vi "Main.vi"(11 "Module Admin":refnum<class "Delacor_lib_QMH_Module Admin.lvclass">) -> ()   [LabVIEW 2021, in "Database.lvlib"]
doc: "This template is based off of the Queued Message Handler design pattern and the Queued Message Handler project template that ships with LabVIEW.\n\nThe main difference is that the queue is private to this module and communication between modules is performed via Broadcast and Request events.\n\nRequest events are wrapped in public API methods and are handled in the Event Handling Loop (EHL) of this VI. Any module can register for Broadcast events sent by this module. The EHL generates messages based on user interface actions.\n\nThe Message Handling Loop (MHL) processes messages generated by the EHL, or by other messages. The messages are string values, so new messages can be added easily to the Message Cases case structure in the MHL. Each message cluster can also provide an optional value for Message Data, which is a variant that can be converted to whatever message-specific data is required.\n_____\nBased on DQMH Project Template 6.1.0.94."
uses:
  Database.lvlib
  <vilib>/Delacor/Delacor QMH/Libraries/Module Admin_class/Delacor_lib_QMH_Module Admin.lvclass
  Class/Access/Access.lvclass
  C:/repository/common_ATE/Libraries/Database/Class/DB/DB.lvclass
  Class/DB/DB.lvclass
  Module Data--cluster.ctl
  <vilib>/Delacor/Delacor QMH/Libraries/Message Queue_class/Delacor_lib_QMH_Message Queue.lvclass/Delacor_lib_QMH_Message Queue.ctl
  Stop Argument--cluster.ctl
  <vilib>/Delacor/Delacor QMH/Libraries/Module Admin_class/Delacor_lib_QMH_Module Admin.lvclass/Delacor_lib_QMH_Module Admin.ctl
  REQ Add User Argument--cluster.ctl
  Class/DB/Credential.ctl
  REQ Check Credential Argument--cluster.ctl
  REQ Check Credential (Reply Payload)--cluster.ctl
  REQ Delete User Argument--cluster.ctl
  REQ Update User Details Argument--cluster.ctl
  Class/DB/Update Credential.ctl
  REQ List Table Argument--cluster.ctl
  REQ List Table (Reply Payload)--cluster.ctl
  REQ Delete Table Data Argument--cluster.ctl
  REQ Save DB Record Data Argument--cluster.ctl
  REQ Save Test Data Argument--cluster.ctl
  REQ Load Test Data Argument--cluster.ctl
  REQ Load Test Data (Reply Payload)--cluster.ctl
  REQ Get Username Argument--cluster.ctl
  REQ Get Username (Reply Payload)--cluster.ctl
  REQ Close DB Ref Argument--cluster.ctl
  <vilib>/Utility/miscctls.llb/LVPointTypeDef.ctl
  <vilib>/Delacor/Delacor QMH/Libraries/Message Queue_class/Delacor_lib_QMH_Enqueue Message (Single).vi
  <vilib>/Delacor/Delacor QMH/Libraries/Module Admin_class/Delacor_lib_QMH_Get External Launch.vi
  <vilib>/Utility/error.llb/Error Cluster From Error Code.vi
  <vilib>/ErrorRing/Error Ring.xnode
  <vilib>/Delacor/Delacor QMH/Libraries/Message Queue_class/Delacor_lib_QMH_Message Queue.lvclass
panel:
  out "error out":errorcluster
  out "Status":string
  in  "Simulate MHL Error":bool
  in  "Simulate EHL Error":bool
  # "Other QMH Modules communicate with this Module via its Public API (wrappers for its Request Events).\n\nThis Module communicates with other Modules via its Broadcast Events.\nAny module that wants to get these messages, just registers for this module's Broadcast events."
  # "This template is for the Delacor Modified Queued Message Handler design pattern.\n\nSee the block diagram for more information on how to use this template."
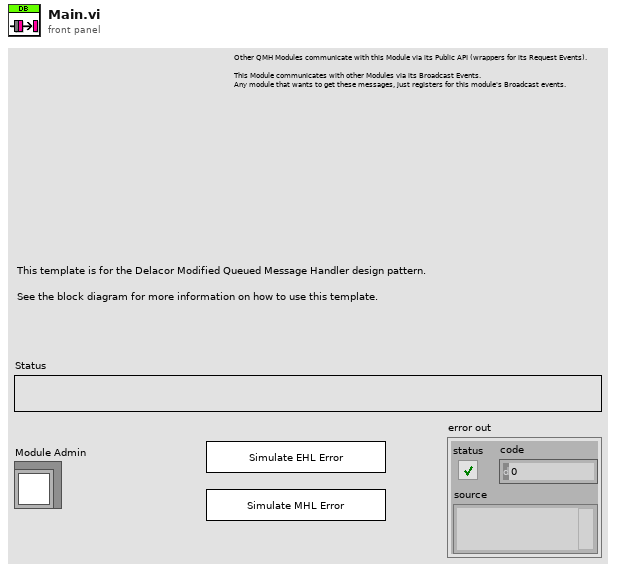
[diagram p1: front panel]
types:
  T1 = typedef "Database.lvlib/Request Events--cluster.ctl" = cluster{"Stop Module":refnum<user-event>, "Show Panel":refnum<user-event>, "Hide Panel":refnum<user-event>, "Get Module Execution Status":refnum<user-event>, "Show Diagram":refnum<user-event>, "REQ Add User":refnum<user-event>, "REQ Check Credential":refnum<user-event>, "REQ Delete User":refnum<user-event>, "REQ Update User Details":refnum<user-event>, "REQ List Table":refnum<user-event>, "REQ Delete Table Data":refnum<user-event>, "REQ Save DB Record Data":refnum<user-event>, "REQ Save Test Data":refnum<user-event>, "REQ Load Test Data":refnum<user-event>, "REQ Get Username":refnum<user-event>, "REQ Close DB Ref":refnum<user-event>}
  T2 = typedef "Database.lvlib/Module Data--cluster.ctl" = cluster{"Status":string, "DB.lvclass":refnum<class "DB.lvclass">}
  T3 = enum32{"invalid lock state", "Not Locked", "Locked (No Password)", "Password-protected"}
  T4 = typedef "Database.lvlib/Stop Argument--cluster.ctl" = cluster{"Origin":string, "Exit via Stop Module Req?":bool, "Wait for Module to stop?":bool}
  T5 = typedef "Database.lvlib/REQ Add User Argument--cluster.ctl" = cluster{"Credential":T6}
  T6 = typedef "Database.lvlib/Credential.ctl" = cluster{"User Level":enum16{"Administrator", "Engineer", "Operator"}, "User Name":string, "Password":string}
  T7 = typedef "Database.lvlib/REQ Check Credential Argument--cluster.ctl" = cluster{"Credential":T6, "Wait Notifier":refnum<notifier>, "wait for reply":bool}
  T8 = typedef "Database.lvlib/REQ Delete User Argument--cluster.ctl" = cluster{"Credential":T6}
  T9 = typedef "Database.lvlib/REQ Update User Details Argument--cluster.ctl" = cluster{"Update Credential":T10}
  T10 = typedef "Database.lvlib/Update Credential.ctl" = cluster{"User Level":enum16{"Administrator", "Engineer", "Operator"}, "User Name":string, "Old Password":string, "New Password":string}
  T11 = typedef "Database.lvlib/REQ List Table Argument--cluster.ctl" = cluster{"Table?":bool, "Wait Notifier":refnum<notifier>, "wait for reply":bool}
  T12 = typedef "Database.lvlib/REQ Delete Table Data Argument--cluster.ctl" = cluster{"Table name":string}
  T13 = typedef "Database.lvlib/REQ Save DB Record Data Argument--cluster.ctl" = cluster{"Boolean":bool}
  T14 = typedef "Database.lvlib/REQ Save Test Data Argument--cluster.ctl" = cluster{"Test Data":string[]}
  T15 = typedef "Database.lvlib/REQ Load Test Data Argument--cluster.ctl" = cluster{"From":timestamp, "To":timestamp, "Wait Notifier":refnum<notifier>, "wait for reply":bool}
  T16 = typedef "Database.lvlib/REQ Get Username Argument--cluster.ctl" = cluster{"User Level":enum16{"Administrator", "Engineer", "Operator"}, "Wait Notifier":refnum<notifier>, "wait for reply":bool}
  T17 = typedef "Database.lvlib/REQ Close DB Ref Argument--cluster.ctl" = cluster{"Boolean":bool}
  T18 = typedef "LVPointTypeDef.ctl" = cluster{"Horizontal":i16, "Vertical":i16}
  T19 = enum32{"Invalid", "Standard", "Closed", "Hidden", "Minimized", "Maximized"}
  T20 = typedef "Database.lvlib/REQ Check Credential (Reply Payload)--cluster.ctl" = cluster{"Match?":bool, "error":errorcluster}
  T21 = typedef "Database.lvlib/REQ List Table (Reply Payload)--cluster.ctl" = cluster{"List Table":string[], "error":errorcluster}
  T22 = typedef "Database.lvlib/REQ Load Test Data (Reply Payload)--cluster.ctl" = cluster{"Test Data":string[][], "error":errorcluster}
  T23 = typedef "Database.lvlib/REQ Get Username (Reply Payload)--cluster.ctl" = cluster{"Username":string[], "error":errorcluster}
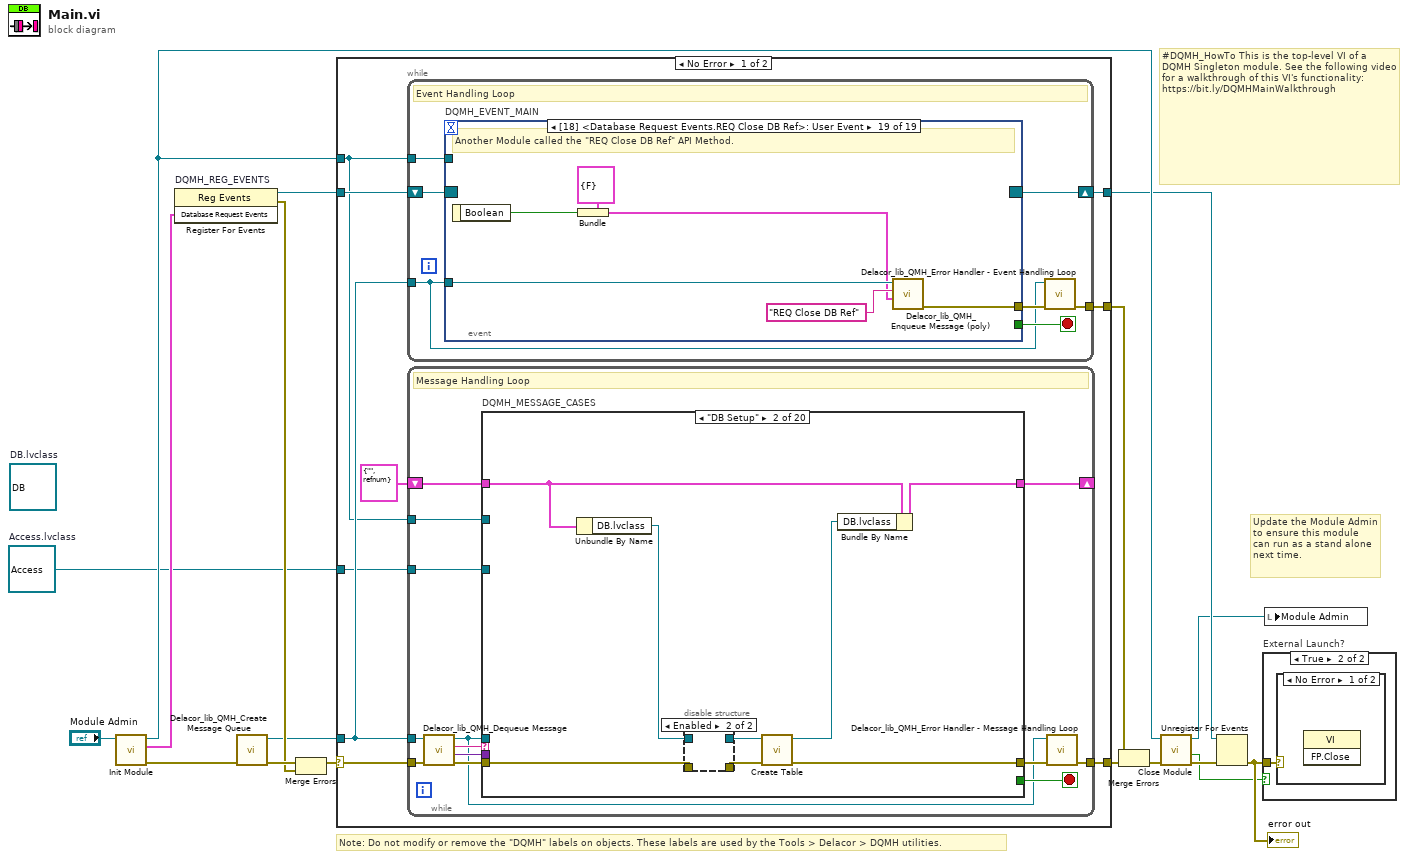
[diagram p0: block diagram]
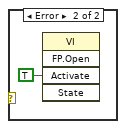
[diagram p3: hidden frame]
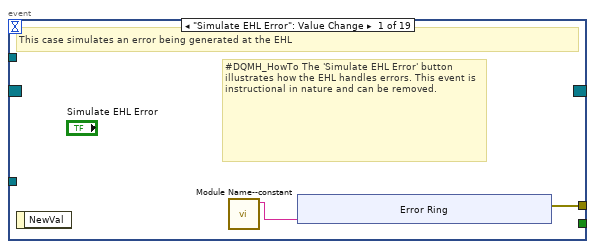
[diagram p4: hidden frame]
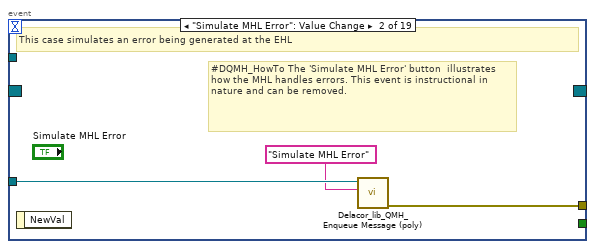
[diagram p5: hidden frame]
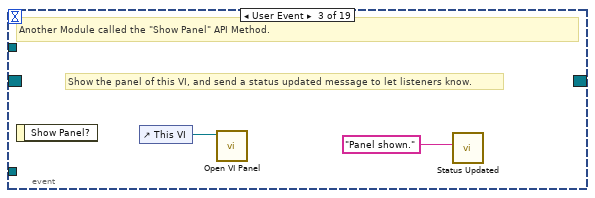
[diagram p6: hidden frame]
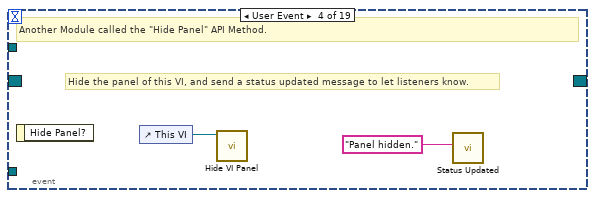
[diagram p7: hidden frame]
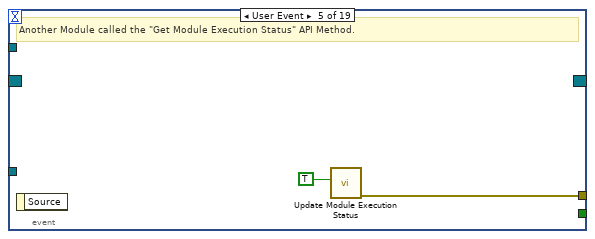
[diagram p8: hidden frame]
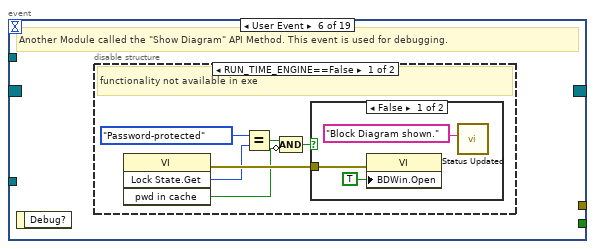
[diagram p9: hidden frame]
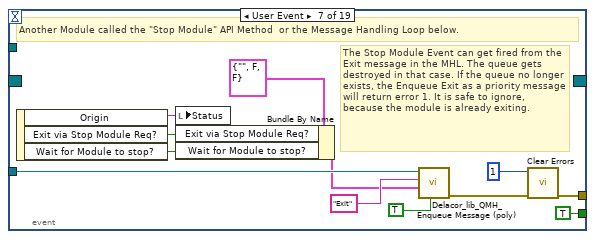
[diagram p12: hidden frame]
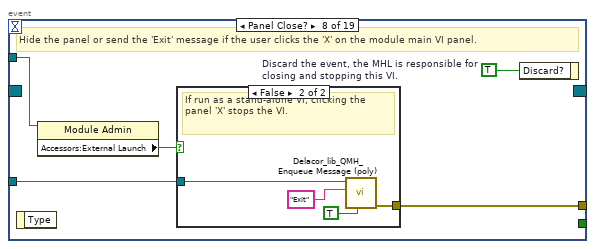
[diagram p13: hidden frame]
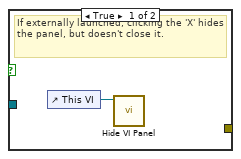
[diagram p14: hidden frame]
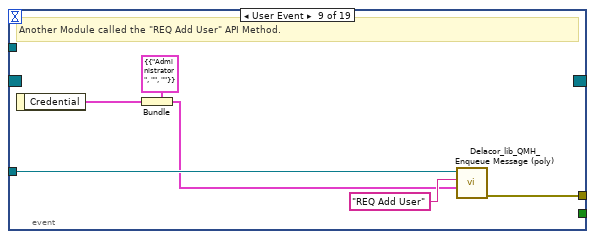
[diagram p15: hidden frame]
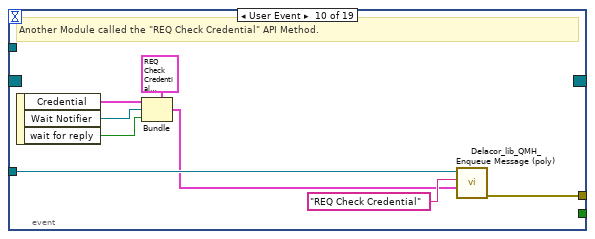
[diagram p16: hidden frame]
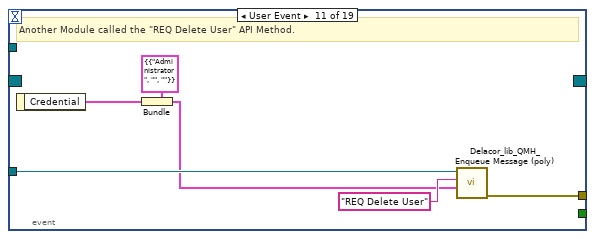
[diagram p17: hidden frame]
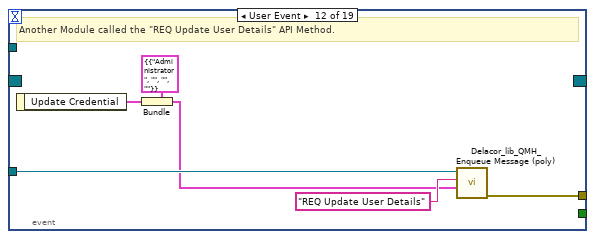
[diagram p18: hidden frame]
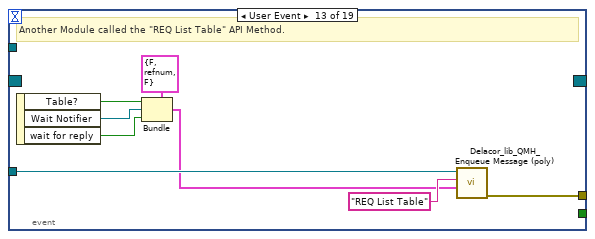
[diagram p19: hidden frame]
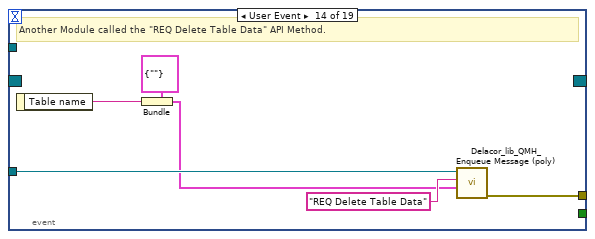
[diagram p20: hidden frame]
diagram:
  w1 = refnum<class "Access.lvclass"> refnum  # Access.lvclass
  (unwired) refnum<class "DB.lvclass"> refnum  # DB.lvclass
  # "#DQMH_HowTo This is the top-level VI of a DQMH Singleton module. See the following video for a walkthrough of this VI's functionality: https://bit.ly/DQMHMainWalkthrough"
  # "Note: Do not modify or remove the \"DQMH\" labels on objects. These labels are used by the Tools > Delacor > DQMH utilities."
  # "Update the Module Admin to ensure this module can run as a stand alone next time."
  n1 = call "Init Module.vi"("Singleton Module Admin in"="Module Admin") -> ("error out"=w17:errorcluster, "Database Request Events"=w6:T1, "Singleton Module Admin out"=w9:refnum<class "Delacor_lib_QMH_Module Admin.lvclass">)  [unwired: 8 in]
  n2 = register-events "DQMH_REG_EVENTS"(w6) -> (reference out=w7:refnum<event-registration>, error out=w10:errorcluster)  [unwired: 2 in]
  n3 = call <vilib>:"Delacor_lib_QMH_Create Message Queue.vi"("error in"=w17) -> ("error out"=w12:errorcluster, "Message Queue"=w5:refnum<class "Delacor_lib_QMH_Message Queue.lvclass">)  [unwired: 9 in]
  n4 = Merge Errors(w12, w10) -> (w11:errorcluster)
  n5 = case shown="No Error" w11 {
    selector: w11 -> [w25 w426]
    tunnel: [w27 w425] -> w18
    tunnel: [w24 w431] -> w8
    tunnel: w7 -> [w22 w431]
    tunnel: w5 -> [w21 w424]
    tunnel: [w26 _] -> w15
    tunnel: w9 -> [w20 w427]
    tunnel: w1 -> [w19 _]
    frame No Error {
      n6 = while {
        tunnel: w21 -> [w28]
        shift-right: [w31] -> w24
        shift-left: w22 -> [w32]
        tunnel: [w33] -> w26
        tunnel: w20 -> [w29]
        stop <- w30 stop-if-true
        # "Event Handling Loop"
        n7 = event "DQMH_EVENT_MAIN" shown="[18] <Database Request Events.REQ Close DB Ref>: User Event" {
          selector: w32 -> [_ _ _ _ _ _ _ _ _ _ _ _ _ _ _ _ _ _ _]
          dyn-events: [_ _ _ _ _ _ _ _ _ _ _ _ _ _ _ _ _ _ _] -> w31
          timeout: _ -> [_ _ _ _ _ _ _ _ _ _ _ _ _ _ _ _ _ _ _]
          tunnel: [_ _ _ _ _ _ TRUE ("Discard?") _ _ _ _ _ _ _ _ _ _ _ _] -> w30
          tunnel: w28 -> [_ w45 _ _ _ _ w69 w76 w89 w97 w103 w109 w117 w123 w129 w135 w144 w152 w158]
          tunnel: [w36 w46 _ _ w52 _ w72 w78 w85 w90 w98 w104 w110 w118 w124 w130 w136 w145 w153] -> w34
          tunnel: w29 -> [_ _ _ _ _ _ _ w75 _ _ _ _ _ _ _ _ _ _ _]
          event "Simulate EHL Error": Value Change {
            # "#DQMH_HowTo The 'Simulate EHL Error' button  illustrates how the EHL handles errors. This event is instructional in nature and can be removed."
            # "This case simulates an error being generated at the EHL"
            n8 = event-data() -> ()  [unwired: 1 in, 1 out]
            n9 = call "Module Name--constant.vi"() -> ("Module Name"=w35:string)  [unwired: 11 in]
            n10 = xnode "Error Ring"("parameter 0"=w35) -> ("error out"=w36:errorcluster)
          }
          event "Simulate MHL Error": Value Change {
            # "#DQMH_HowTo The 'Simulate MHL Error' button  illustrates how the MHL handles errors. This event is instructional in nature and can be removed."
            # "This case simulates an error being generated at the EHL"
            n11 = event-data() -> ()  [unwired: 1 in, 1 out]
            n12 = call-poly <vilib>:"Delacor_lib_QMH_Enqueue Message (poly).vi"("Message"="Simulate MHL Error", "Message Queue in"=w45) -> ("error out"=w46:errorcluster)  [unwired: 8 in, 1 out]
          }
          event User Event {
            # "Show the panel of this VI, and send a status updated message to let listeners know."
            # "Another Module called the \"Show Panel\" API Method."
            n13 = event-data() -> ()  [unwired: 1 in, 1 out]
            n14 = control-ref of="This VI"() -> (w48:refnum<vi>)
            n15 = call "Open VI Panel.vi"("VI"=w48) -> ()  [unwired: 10 in, 1 out]
            n16 = call "Status Updated.vi"("Status"="Panel shown." ("format string")) -> ()  [unwired: 10 in, 1 out]
          }
          event User Event {
            # "Hide the panel of this VI, and send a status updated message to let listeners know."
            # "Another Module called the \"Hide Panel\" API Method."
            n17 = event-data() -> ()  [unwired: 1 in, 1 out]
            n18 = control-ref of="This VI"() -> (w50:refnum<vi>)
            n19 = call "Hide VI Panel.vi"("VI"=w50) -> ()  [unwired: 10 in, 1 out]
            n20 = call "Status Updated.vi"("Status"="Panel hidden." ("format string")) -> ()  [unwired: 10 in, 1 out]
          }
          event User Event {
            # "Another Module called the \"Get Module Execution Status\" API Method."
            n21 = event-data() -> ()  [unwired: 1 in, 1 out]
            n22 = call "Update Module Execution Status.vi"("Running?"=TRUE) -> ("error out"=w52:errorcluster)  [unwired: 10 in]
          }
          event User Event {
            # "Another Module called the \"Show Diagram\" API Method. This event is used for debugging."
            n23 = event-data() -> ()  [unwired: 1 in, 1 out]
            n24 = disable-structure shown="RUN_TIME_ENGINE==False" {
              frame condition #0 (active) {
                # "functionality not available in exe"
                n25 = invoke class="VI" method="Lock State.Get"() -> (error out=w58:errorcluster, "Get Lock State"=w57:T3, "pwd in cache"=w54:bool)  [unwired: 4 in, 1 out]
                n26 = Equal?(x=T3."Password-protected", y=w57) -> (x = y?=w55:bool)
                n27 = Compound Arithmetic op=AND(w55, invert w54) -> (w53:bool)
                n28 = case shown="False" w53 {
                  tunnel: w58 -> [w61 _]
                  frame False {
                    n29 = property class="VI"(error in=w61, "BDWin.Open"=TRUE ("Block Diagram Window:Open")) -> ()  [unwired: 1 in, 2 out]
                    n30 = call "Status Updated.vi"("Status"="Block Diagram shown." ("format string")) -> ()  [unwired: 10 in, 1 out]
                  }
                  frame True {
                    # "Password-protected VI, and the password is not in the cache. Do not show the diagram."
                  }
                }
              }
              frame condition #1 {
              }
            }
          }
          event User Event {
            # "The Stop Module Event can get fired from the Exit message in the MHL. The queue gets destroyed in that case. If the queue no longer exists, the Enqueue Exit as a priority message will return error 1. It is safe to ignore, because the module is already exiting."
            # "Another Module called the \"Stop Module\" API Method  or the Message Handling Loop below."
            n31 = event-data() -> ("Origin"=w68:string, "Exit via Stop Module Req?"=w64:bool, "Wait for Module to stop?"=w63:bool)  [unwired: 1 in]
            n32 = local write "Status"(w68) -> ()
            n33 = Bundle By Name(cluster=T4 {"Origin"="", "Exit via Stop Module Req?"=FALSE, "Wait for Module to stop?"=FALSE} ("Stop Argument"), "Exit via Stop Module Req?"=w64, "Wait for Module to stop?"=w63) -> (w62:T4)
            n34 = call-poly <vilib>:"Delacor_lib_QMH_Enqueue Message (poly).vi"("Priority Message? (F)"=TRUE, "Message Data"=w62, "Message"="Exit", "Message Queue in"=w69) -> ("error out"=w73:errorcluster)  [unwired: 6 in, 1 out]
            n35 = call <vilib>:"Clear Errors.vi"("error in (no error)"=w73, "specific error code to clear (0: all)"=1) -> ("error out"=w72:errorcluster)  [unwired: 4 in, 1 out]
          }
          event Panel Close? {
            w77 = TRUE  # Discard the event, the MHL is responsible for closing and stopping this VI.
            # "Hide the panel or send the 'Exit' message if the user clicks the 'X' on the module main VI panel."
            n36 = event-data() -> ()  [unwired: 1 in, 1 out]
            n37 = property class="Module Admin"(reference=w75) -> ("Accessors:External Launch"=w74:bool)  [unwired: 1 in, 2 out]
            n38 = case shown="False" w74 {
              tunnel: w76 -> [_ w82]
              tunnel: [_ w83] -> w78
              frame True {
                # "If externally launched, clicking the 'X' hides the panel, but doesn't close it."
                n39 = control-ref of="This VI"() -> (w79:refnum<vi>)
                n40 = call "Hide VI Panel.vi"("VI"=w79) -> ()  [unwired: 10 in, 1 out]
              }
              frame False {
                # "If run as a stand-alone VI, clicking the panel 'X' stops the VI."
                n41 = call-poly <vilib>:"Delacor_lib_QMH_Enqueue Message (poly).vi"("Priority Message? (F)"=TRUE, "Message"="Exit", "Message Queue in"=w82) -> ("error out"=w83:errorcluster)  [unwired: 7 in, 1 out]
              }
            }
            n42 = event-data("Discard?"=w77) -> ()  [unwired: 1 in, 1 out]
          }
          event User Event {
            # "Another Module called the \"REQ Add User\" API Method."
            n43 = event-data() -> ("Credential"=w84:T6)  [unwired: 1 in]
            n44 = Bundle(cluster=T5 {"Credential"={"User Level"=enum."Administrator", "User Name"="", "Password"=""}} ("REQ Add User Argument"), "Credential"=w84) -> (w86:T5)
            n45 = call-poly <vilib>:"Delacor_lib_QMH_Enqueue Message (poly).vi"("Message Data"=w86, "Message"="REQ Add User", "Message Queue in"=w89) -> ("error out"=w85:errorcluster)  [unwired: 7 in, 1 out]
          }
          event User Event {
            # "Another Module called the \"REQ Check Credential\" API Method."
            n46 = event-data() -> ("Credential"=w93:T6, "Wait Notifier"=w92:refnum<notifier>, "wait for reply"=w91:bool)  [unwired: 1 in]
            n47 = Bundle(cluster=T7 {"Credential"={"User Level"=enum."Administrator", "User Name"="", "Password"=""}, "Wait Notifier"=refnum, "wait for reply"=FALSE} ("REQ Check Credential Argument"), "Credential"=w93, "Wait Notifier"=w92, "wait for reply"=w91) -> (w94:T7)
            n48 = call-poly <vilib>:"Delacor_lib_QMH_Enqueue Message (poly).vi"("Message Data"=w94, "Message"="REQ Check Credential", "Message Queue in"=w97) -> ("error out"=w90:errorcluster)  [unwired: 7 in, 1 out]
          }
          event User Event {
            # "Another Module called the \"REQ Delete User\" API Method."
            n49 = event-data() -> ("Credential"=w99:T6)  [unwired: 1 in]
            n50 = Bundle(cluster=T8 {"Credential"={"User Level"=enum."Administrator", "User Name"="", "Password"=""}} ("REQ Delete User Argument"), "Credential"=w99) -> (w100:T8)
            n51 = call-poly <vilib>:"Delacor_lib_QMH_Enqueue Message (poly).vi"("Message Data"=w100, "Message"="REQ Delete User", "Message Queue in"=w103) -> ("error out"=w98:errorcluster)  [unwired: 7 in, 1 out]
          }
          event User Event {
            # "Another Module called the \"REQ Update User Details\" API Method."
            n52 = event-data() -> ("Update Credential"=w105:T10)  [unwired: 1 in]
            n53 = Bundle(cluster=T9 {"Update Credential"={"User Level"=enum."Administrator", "User Name"="", "Old Password"="", "New Password"=""}} ("REQ Update User Details Argument"), "Update Credential"=w105) -> (w106:T9)
            n54 = call-poly <vilib>:"Delacor_lib_QMH_Enqueue Message (poly).vi"("Message Data"=w106, "Message"="REQ Update User Details", "Message Queue in"=w109) -> ("error out"=w104:errorcluster)  [unwired: 7 in, 1 out]
          }
          event User Event {
            # "Another Module called the \"REQ List Table\" API Method."
            n55 = event-data() -> ("Table?"=w113:bool, "Wait Notifier"=w112:refnum<notifier>, "wait for reply"=w111:bool)  [unwired: 1 in]
            n56 = Bundle(cluster=T11 {"Table?"=FALSE, "Wait Notifier"=refnum, "wait for reply"=FALSE} ("REQ List Table Argument"), "Table?"=w113, "Wait Notifier"=w112, "wait for reply"=w111) -> (w114:T11)
            n57 = call-poly <vilib>:"Delacor_lib_QMH_Enqueue Message (poly).vi"("Message Data"=w114, "Message"="REQ List Table", "Message Queue in"=w117) -> ("error out"=w110:errorcluster)  [unwired: 7 in, 1 out]
          }
          event User Event {
            # "Another Module called the \"REQ Delete Table Data\" API Method."
            n58 = event-data() -> ("Table name"=w119:string)  [unwired: 1 in]
            n59 = Bundle(cluster=T12 {"Table name"=""} ("REQ Delete Table Data Argument"), "Table name"=w119) -> (w120:T12)
            n60 = call-poly <vilib>:"Delacor_lib_QMH_Enqueue Message (poly).vi"("Message Data"=w120, "Message"="REQ Delete Table Data", "Message Queue in"=w123) -> ("error out"=w118:errorcluster)  [unwired: 7 in, 1 out]
          }
          event User Event {
            # "Another Module called the \"REQ Save DB Record Data\" API Method."
            n61 = event-data() -> ("Boolean"=w125:bool)  [unwired: 1 in]
            n62 = Bundle(cluster=T13 {"Boolean"=FALSE} ("REQ Save DB Record Data Argument"), "Boolean"=w125) -> (w126:T13)
            n63 = call-poly <vilib>:"Delacor_lib_QMH_Enqueue Message (poly).vi"("Message Data"=w126, "Message"="REQ Save DB Record Data", "Message Queue in"=w129) -> ("error out"=w124:errorcluster)  [unwired: 7 in, 1 out]
          }
          event User Event {
            # "Another Module called the \"REQ Save Test Data\" API Method."
            n64 = event-data() -> ("Test Data"=w131:string[])  [unwired: 1 in]
            n65 = Bundle(cluster=T14 {"Test Data"=[]} ("REQ Save Test Data Argument"), "Test Data"=w131) -> (w132:T14)
            n66 = call-poly <vilib>:"Delacor_lib_QMH_Enqueue Message (poly).vi"("Message Data"=w132, "Message"="REQ Save Test Data", "Message Queue in"=w135) -> ("error out"=w130:errorcluster)  [unwired: 7 in, 1 out]
          }
          event User Event {
            # "Another Module called the \"REQ Load Test Data\" API Method."
            n67 = event-data() -> ("From"=w140:timestamp, "To"=w139:timestamp, "Wait Notifier"=w138:refnum<notifier>, "wait for reply"=w137:bool)  [unwired: 1 in]
            n68 = Bundle(cluster=T15 {"From"=timestamp(0 s since 1904-01-01), "To"=timestamp(0 s since 1904-01-01), "Wait Notifier"=refnum, "wait for reply"=FALSE} ("REQ Load Test Data Argument"), "From"=w140, "To"=w139, "Wait Notifier"=w138, "wait for reply"=w137) -> (w141:T15)
            n69 = call-poly <vilib>:"Delacor_lib_QMH_Enqueue Message (poly).vi"("Message Data"=w141, "Message"="REQ Load Test Data", "Message Queue in"=w144) -> ("error out"=w136:errorcluster)  [unwired: 7 in, 1 out]
          }
          event User Event {
            # "Another Module called the \"REQ Get Username\" API Method."
            n70 = event-data() -> ("User Level"=w148:enum16{"Administrator", "Engineer", "Operator"}, "Wait Notifier"=w147:refnum<notifier>, "wait for reply"=w146:bool)  [unwired: 1 in]
            n71 = Bundle(cluster=T16 {"User Level"=enum."Administrator", "Wait Notifier"=refnum, "wait for reply"=FALSE} ("REQ Get Username Argument"), "User Level"=w148, "Wait Notifier"=w147, "wait for reply"=w146) -> (w149:T16)
            n72 = call-poly <vilib>:"Delacor_lib_QMH_Enqueue Message (poly).vi"("Message Data"=w149, "Message"="REQ Get Username", "Message Queue in"=w152) -> ("error out"=w145:errorcluster)  [unwired: 7 in, 1 out]
          }
          event User Event {
            # "Another Module called the \"REQ Close DB Ref\" API Method."
            n73 = event-data() -> ("Boolean"=w154:bool)  [unwired: 1 in]
            n74 = Bundle(cluster=T17 {"Boolean"=FALSE} ("REQ Close DB Ref Argument"), "Boolean"=w154) -> (w155:T17)
            n75 = call-poly <vilib>:"Delacor_lib_QMH_Enqueue Message (poly).vi"("Message Data"=w155, "Message"="REQ Close DB Ref", "Message Queue in"=w158) -> ("error out"=w153:errorcluster)  [unwired: 7 in, 1 out]
          }
        }
        n76 = call-dynamic "Delacor_lib_QMH_Error Handler - Event Handling Loop.vi"("error in"=w34, "Message Queue in"=w28) -> ("dup error in"=w33:errorcluster)  [unwired: 8 in, 1 out]
      }
      n77 = while {
        tunnel: w21 -> [w162]
        shift-right: [w166] -> _
        shift-left: T2 {"Status"="", "DB.lvclass"=refnum} ("Data Cluster") -> [w167]
        tunnel: w25 -> [w170]
        tunnel: [w168] -> w27
        tunnel: w20 -> [w160]
        tunnel: w19 -> [w159]
        stop <- w165 stop-if-true
        # "Message Handling Loop"
        n78 = call-dynamic "Delacor_lib_QMH_Dequeue Message.vi"("error in"=w170, "Message Queue in"=w162) -> ("error out"=w169:errorcluster, "Message Data"=w163:variant, "Message"=w164:string, "Message Queue out"=w161:refnum<class "Delacor_lib_QMH_Message Queue.lvclass">)  [unwired: 6 in]
        n79 = case "DQMH_MESSAGE_CASES" shown="\"DB Setup\"" w164 {
          selector: w164 -> [_ _ _ _ _ _ _ _ _ _ _ _ _ _ _ _ _ _ _ w411]
          tunnel: w161 -> [w172 _ _ _ _ _ _ _ _ _ _ _ _ _ _ _ _ w379 w404 _]
          tunnel: w169 -> [w193 w203 w223 w236 w254 w265 w280 w293 w299 w310 w327 w345 w357 w359 w362 w364 w369 w386 w409 w413]
          tunnel: [w173 w198 w214 w226 w249 w260 w271 w288 w297 w305 w318 w331 w353 w359 w361 w364 w368 w382 w406 w414] -> w171
          tunnel: w167 -> [w183 w202 w213 w230 w248 w259 w269 w286 w298 w304 w317 w336 w352 w358 w360 w363 w366 w381 w395 w412]
          tunnel: [w182 w197 w211 w228 w246 w256 w267 w284 w298 w302 w315 w334 w350 w358 w360 w363 w366 w381 w395 w412] -> w166
          tunnel: [_ _ _ _ _ _ _ _ _ _ _ _ _ _ _ _ _ _ w403 _] -> w165
          tunnel: w163 -> [_ _ w222 w235 w253 w264 w279 w292 w296 w309 w326 w344 w356 _ _ _ _ w380 w402 _]
          tunnel: w160 -> [w184 _ _ _ _ _ _ _ _ _ _ _ _ _ _ _ _ w378 w397 _]
          tunnel: w159 -> [w176 _ _ _ _ _ _ _ _ _ _ _ _ _ _ _ _ _ _ _]
          frame "Initialize" {
            w178 = "Initial Message" ("Initial Message")
            # "Initialize - Any operation that needs to be done before the module can receive messages. Synchronize Caller Events.vi will inform Start Module.vi that the module has launched and is ready to receive messages. Module Did Init.vi will broadcast that the module initialized."
            n80 = call "Synchronize Caller Events.vi"("error in (no error)"=w193, "Singleton Module Admin in"=w184) -> ("error out"=w192:errorcluster, "Singleton Module Admin out"=w179:refnum<class "Delacor_lib_QMH_Module Admin.lvclass">)  [unwired: 8 in]
            n81 = property class="Module Admin"(reference=w179) -> ("Accessors:External Launch"=w188:bool)  [unwired: 1 in, 2 out]
            n82 = Select(t=T19."Hidden" ("State"), s=w188, f=T19."Standard" ("State")) -> (s? t:f=w185:T19)
            n83 = call "Module Name--constant.vi"() -> ("Module Name"=w180:string)  [unwired: 11 in]
            n84 = call "Module Name--constant.vi"() -> ("Module Name"=w191:string)  [unwired: 11 in]
            n85 = property class="VI"("Front Panel.Title"=w191) -> (reference out=w190:refnum<vi>, error out=w195:errorcluster)  [unwired: 2 in]
            n86 = call "Module Did Init.vi"("error in (no error)"=w192, "Initialized?"=TRUE, "Origin"=w180) -> ("error out"=w174:errorcluster)  [unwired: 8 in]
            n87 = invoke class="VI" method="FP.Open"(reference=w190, error in=w195, "State"=w185) -> (reference out=w189:refnum<vi>, error out=w194:errorcluster)  [unwired: 2 in, 3 out]
            n88 = Bundle By Name(cluster=w183, "Status"=w178, "DB.lvclass"=w176) -> (w182:T2)
            n89 = call-poly <vilib>:"Delacor_lib_QMH_Enqueue Message (poly).vi"("error in"=w174, "Message"="DB Setup", "Message Queue in"=w172) -> ("error out"=w173:errorcluster)  [unwired: 7 in, 1 out]
            n90 = invoke class="VI" method="FP.Center"(reference=w189, error in=w194) -> ()  [unwired: 1 in, 3 out]
            n91 = property on="Pane" class="Pane"("Origin"=T18 {"Horizontal"=0, "Vertical"=0}) -> ()  [unwired: 2 in, 2 out]
            "Status" <- w178
          }
          frame "DB Setup" {
            n92 = Unbundle By Name(w202) -> ("DB.lvclass"=w201:refnum<class "DB.lvclass">)
            n93 = disable-structure shown="Enabled" {
              disable-tunnel: w203 -> [w207 _]
              disable-tunnel: w201 -> [w206 _]
              disable-tunnel: [w205 _] -> w200
              disable-tunnel: [w204 _] -> w199
              frame Disabled {
                n94 = call-dynamic "Open DB Ref.vi"("error in (no error)"=w207, "DB in"=w206) -> ("error out"=w205:errorcluster, "DB out"=w204:refnum<class "DB.lvclass">)  [unwired: 8 in]
              }
              frame Enabled {
              }
            }
            n95 = call-dynamic "Create Table.vi"("error in (no error)"=w200, "DB in"=w199) -> ("error out"=w198:errorcluster, "DB out"=w196:refnum<class "DB.lvclass">)  [unwired: 8 in]
            n96 = Bundle By Name(cluster=w202, "DB.lvclass"=w196) -> (w197:T2)
          }
          frame "REQ Check Credential" {
            n97 = Variant To Data(error in=w223, type=T7 {"Credential"={"User Level"=enum."Administrator", "User Name"="", "Password"=""}, "Wait Notifier"=refnum, "wait for reply"=FALSE} ("REQ Check Credential Argument"), Variant=w222) -> (data=w220:T7, error out=w215:errorcluster)
            n98 = Unbundle By Name(w220) -> ("Wait Notifier"=w219:refnum<notifier>, "wait for reply"=w218:bool, "Credential"=w209:T6)
            n99 = Unbundle By Name(w213) -> ("DB.lvclass"=w212:refnum<class "DB.lvclass">)
            n100 = call-dynamic "Check Credential.vi"("error in (no error)"=w215, "Credential"=w209, "DB in"=w212) -> ("error out"=w214:errorcluster, "Match?"=w208:bool, "DB out"=w210:refnum<class "DB.lvclass">)  [unwired: 6 in]
            n101 = Bundle By Name(cluster=w213, "DB.lvclass"=w210) -> (w211:T2)
            n102 = Bundle By Name(cluster=T20 {"Match?"=FALSE, "error"={"status"=FALSE, "code"=0, "source"=""}} ("REQ Check Credential (Reply Payload)"), "Match?"=w208) -> (w217:T20)
            n103 = case "DQMH_FIRE_NOTIFIER" shown="True" w218 {
              tunnel: w219 -> [_ w225]
              tunnel: w217 -> [_ w224]
              frame False {
              }
              frame True {
                n104 = Send Notification(notification=w224, notifier=w225) -> ()  [unwired: 1 in, 2 out]
              }
            }
          }
          frame "REQ Add User" {
            n105 = Variant To Data(error in=w236, type=T5 {"Credential"={"User Level"=enum."Administrator", "User Name"="", "Password"=""}} ("REQ Add User Argument"), Variant=w235) -> (data=w233:T5, error out=w232:errorcluster)
            n106 = Unbundle By Name(w233) -> ("Credential"=w231:T6)
            n107 = Unbundle By Name(w230) -> ("DB.lvclass"=w229:refnum<class "DB.lvclass">)
            n108 = disable-structure shown="Enabled" {
              disable-tunnel: w232 -> [w241 w242]
              disable-tunnel: w231 -> [w240 _]
              disable-tunnel: w229 -> [w239 w243]
              disable-tunnel: [w238 w243] -> w227
              disable-tunnel: [w237 w242] -> w226
              frame Disabled {
                n109 = call-dynamic "Add User.vi"("error in (no error)"=w241, "Credential"=w240, "DB in"=w239) -> ("error out"=w237:errorcluster, "DB out"=w238:refnum<class "DB.lvclass">)  [unwired: 7 in]
              }
              frame Enabled {
              }
            }
            n110 = Bundle By Name(cluster=w230, "DB.lvclass"=w227) -> (w228:T2)
          }
          frame "REQ Delete User" {
            n111 = Variant To Data(error in=w254, type=T8 {"Credential"={"User Level"=enum."Administrator", "User Name"="", "Password"=""}} ("REQ Delete User Argument"), Variant=w253) -> (data=w251:T8, error out=w250:errorcluster)
            n112 = Unbundle By Name(w251) -> ("Credential"=w244:T6)
            n113 = Unbundle By Name(w248) -> ("DB.lvclass"=w247:refnum<class "DB.lvclass">)
            n114 = call-dynamic "Delete User.vi"("error in (no error)"=w250, "Credential"=w244, "DB in"=w247) -> ("error out"=w249:errorcluster, "DB out"=w245:refnum<class "DB.lvclass">)  [unwired: 7 in]
            n115 = Bundle By Name(cluster=w248, "DB.lvclass"=w245) -> (w246:T2)
          }
          frame "REQ Update User Details" {
            n116 = Variant To Data(error in=w265, type=T9 {"Update Credential"={"User Level"=enum."Administrator", "User Name"="", "Old Password"="", "New Password"=""}} ("REQ Update User Details Argument"), Variant=w264) -> (data=w262:T9, error out=w261:errorcluster)
            n117 = Unbundle By Name(w262) -> ("Update Credential"=w257:T10)
            n118 = Unbundle By Name(w259) -> ("DB.lvclass"=w258:refnum<class "DB.lvclass">)
            n119 = call-dynamic "Update User Details.vi"("error in (no error)"=w261, "Update Credential"=w257, "DB in"=w258) -> ("error out"=w260:errorcluster, "DB out"=w255:refnum<class "DB.lvclass">)  [unwired: 7 in]
            n120 = Bundle By Name(cluster=w259, "DB.lvclass"=w255) -> (w256:T2)
          }
          frame "REQ List Table" {
            n121 = Variant To Data(error in=w280, type=T11 {"Table?"=FALSE, "Wait Notifier"=refnum, "wait for reply"=FALSE} ("REQ List Table Argument"), Variant=w279) -> (data=w277:T11, error out=w272:errorcluster)
            n122 = Unbundle By Name(w277) -> ("Wait Notifier"=w276:refnum<notifier>, "wait for reply"=w275:bool)
            n123 = Unbundle By Name(w269) -> ("DB.lvclass"=w268:refnum<class "DB.lvclass">)
            n124 = call-dynamic "List Table.vi"("error in (no error)"=w272, "DB in"=w268) -> ("error out"=w271:errorcluster, "List Table"=w270:string[], "DB out"=w266:refnum<class "DB.lvclass">)  [unwired: 7 in]
            n125 = Bundle By Name(cluster=w269, "DB.lvclass"=w266) -> (w267:T2)
            n126 = Bundle By Name(cluster=T21 {"List Table"=[], "error"={"status"=FALSE, "code"=0, "source"=""}} ("REQ List Table (Reply Payload)"), "List Table"=w270) -> (w274:T21)
            n127 = case "DQMH_FIRE_NOTIFIER" shown="True" w275 {
              tunnel: w276 -> [_ w282]
              tunnel: w274 -> [_ w281]
              frame False {
              }
              frame True {
                n128 = Send Notification(notification=w281, notifier=w282) -> ()  [unwired: 1 in, 2 out]
              }
            }
          }
          frame "REQ Delete Table Data" {
            n129 = Variant To Data(error in=w293, type=T12 {"Table name"=""} ("REQ Delete Table Data Argument"), Variant=w292) -> (data=w290:T12, error out=w289:errorcluster)
            n130 = Unbundle By Name(w290) -> ("Table name"=w287:string)
            n131 = Unbundle By Name(w286) -> ("DB.lvclass"=w285:refnum<class "DB.lvclass">)
            n132 = call-dynamic "Delete Table Data.vi"("error in (no error)"=w289, "Table name"=w287, "DB in"=w285) -> ("error out"=w288:errorcluster, "DB out"=w283:refnum<class "DB.lvclass">)  [unwired: 7 in]
            n133 = Bundle By Name(cluster=w286, "DB.lvclass"=w283) -> (w284:T2)
          }
          frame "REQ Save DB Record Data" {
            n134 = Variant To Data(error in=w299, type=T13 {"Boolean"=FALSE} ("REQ Save DB Record Data Argument"), Variant=w296) -> (data=w294:T13, error out=w297:errorcluster)
            n135 = Unbundle By Name(w294) -> ()  [unwired: 1 out]
          }
          frame "REQ Save Test Data" {
            n136 = Variant To Data(error in=w310, type=T14 {"Test Data"=[]} ("REQ Save Test Data Argument"), Variant=w309) -> (data=w307:T14, error out=w306:errorcluster)
            n137 = Unbundle By Name(w307) -> ("Test Data"=w300:string[])
            n138 = Unbundle By Name(w304) -> ("DB.lvclass"=w303:refnum<class "DB.lvclass">)
            n139 = call-dynamic "Save Test Data.vi"("error in (no error)"=w306, "Test Data"=w300, "DB in"=w303) -> ("error out"=w305:errorcluster, "DB out"=w301:refnum<class "DB.lvclass">)  [unwired: 7 in]
            n140 = Bundle By Name(cluster=w304, "DB.lvclass"=w301) -> (w302:T2)
          }
          frame "REQ Load Test Data" {
            n141 = Variant To Data(error in=w327, type=T15 {"From"=timestamp(0 s since 1904-01-01), "To"=timestamp(0 s since 1904-01-01), "Wait Notifier"=refnum, "wait for reply"=FALSE} ("REQ Load Test Data Argument"), Variant=w326) -> (data=w324:T15, error out=w319:errorcluster)
            n142 = Unbundle By Name(w324) -> ("From"=w312:timestamp, "To"=w311:timestamp, "Wait Notifier"=w323:refnum<notifier>, "wait for reply"=w322:bool)
            n143 = Unbundle By Name(w317) -> ("DB.lvclass"=w316:refnum<class "DB.lvclass">)
            n144 = call-dynamic "Load Test Data.vi"("error in (no error)"=w319, "To"=w311, "From"=w312, "DB in"=w316) -> ("error out"=w318:errorcluster, "Test Data Out"=w313:string[][], "DB out"=w314:refnum<class "DB.lvclass">)  [unwired: 5 in]
            n145 = Bundle By Name(cluster=w317, "DB.lvclass"=w314) -> (w315:T2)
            n146 = Bundle By Name(cluster=T22 {"Test Data"=[], "error"={"status"=FALSE, "code"=0, "source"=""}} ("REQ Load Test Data (Reply Payload)"), "Test Data"=w313) -> (w321:T22)
            n147 = case "DQMH_FIRE_NOTIFIER" shown="True" w322 {
              tunnel: w323 -> [_ w329]
              tunnel: w321 -> [_ w328]
              frame False {
              }
              frame True {
                n148 = Send Notification(notification=w328, notifier=w329) -> ()  [unwired: 1 in, 2 out]
              }
            }
          }
          frame "REQ Get Username" {
            n149 = Variant To Data(error in=w345, type=T16 {"User Level"=enum."Administrator", "Wait Notifier"=refnum, "wait for reply"=FALSE} ("REQ Get Username Argument"), Variant=w344) -> (data=w342:T16, error out=w337:errorcluster)
            n150 = Unbundle By Name(w342) -> ("Wait Notifier"=w341:refnum<notifier>, "wait for reply"=w340:bool, "User Level"=w330:enum16{"Administrator", "Engineer", "Operator"})
            n151 = Unbundle By Name(w336) -> ("DB.lvclass"=w335:refnum<class "DB.lvclass">)
            n152 = call-dynamic "Get Username.vi"("error in (no error)"=w337, "User Level"=w330, "DB in"=w335) -> ("error out"=w331:errorcluster, "Username"=w332:string[], "DB out"=w333:refnum<class "DB.lvclass">)  [unwired: 6 in]
            n153 = Bundle By Name(cluster=w336, "DB.lvclass"=w333) -> (w334:T2)
            n154 = Bundle By Name(cluster=T23 {"Username"=[], "error"={"status"=FALSE, "code"=0, "source"=""}} ("REQ Get Username (Reply Payload)"), "Username"=w332) -> (w339:T23)
            n155 = case "DQMH_FIRE_NOTIFIER" shown="True" w340 {
              tunnel: w341 -> [_ w347]
              tunnel: w339 -> [_ w346]
              frame False {
              }
              frame True {
                n156 = Send Notification(notification=w346, notifier=w347) -> ()  [unwired: 1 in, 2 out]
              }
            }
          }
          frame "REQ Close DB Ref" {
            n157 = Variant To Data(error in=w357, type=T17 {"Boolean"=FALSE} ("REQ Close DB Ref Argument"), Variant=w356) -> (error out=w354:errorcluster)  [unwired: 1 out]
            n158 = Unbundle By Name(w352) -> ("DB.lvclass"=w351:refnum<class "DB.lvclass">)
            n159 = call <vilib>:"Clear Errors.vi"("error in (no error)"=w354) -> ("error out"=w348:errorcluster)  [unwired: 5 in, 1 out]
            n160 = call-dynamic "Close DB Reference.vi"("error in (no error)"=w348, "DB in"=w351) -> ("error out"=w353:errorcluster, "DB out"=w349:refnum<class "DB.lvclass">)  [unwired: 8 in]
            n161 = Bundle By Name(cluster=w352, "DB.lvclass"=w349) -> (w350:T2)
          }
          frame "---Module Specific---" {
            # "Separator -- The following cases handle messages specific to this Module."
          }
          frame "---Copy This Frame---" {
            # "Duplicate this frame when creating new messages.  Change this comment in the duplicated frame to describe this message."
            n162 = Merge Errors(w362) -> (w361:errorcluster)
          }
          frame "---Exit and Error Handling---" {
            # "Separator - The following cases handle errors and exit messages."
          }
          frame "Simulate MHL Error" {
            # "#DQMH_HowTo The 'Simulate MHL Error' button  illustrates how the MHL handles errors. This event is instructional in nature and can be removed."
            # "Simulate an error occurring at the MHL"
            n163 = call "Module Name--constant.vi"() -> ("Module Name"=w365:string)  [unwired: 11 in]
            n164 = xnode "Error Ring"("parameter 0"=w365) -> ("error out"=w367:errorcluster)
            n165 = Merge Errors(w369, w367) -> (w368:errorcluster)
          }
          frame "Error" {
            # "#CodeRecommended - If you ever change the name of this \"Error\" message, you'll need to update the name in the Check Loop Error.vi as well."
            # "#CodeRecommended - If the module is running in standalone mode (External Launch = FALSE), this code will pop up an error dialog and call the 'Exit' message if an error occurs. Add more fine-grained error handling here."
            # "Error - Check the error message data and respond accordingly. This message is sent by the \"Error Handler\" VIs at the end of each loop in this application."
            n166 = property class="Module Admin"(reference=w378) -> ("Accessors:External Launch"=w377:bool)  [unwired: 1 in, 2 out]
            n167 = Variant To Data(error in=w386, type=errorcluster {"status"=FALSE, "code"=0, "source"=""} ("error constant"), Variant=w380) -> (data=w387:errorcluster, error out=w384:errorcluster)
            n168 = call "Error Reported.vi"("Error"=w387) -> ()  [unwired: 10 in, 1 out]
            n169 = case shown="False" w377 {
              tunnel: [w392 _] -> w383
              tunnel: w379 -> [w390 _]
              tunnel: w387 -> [w391 _]
              frame False {
                # "If the module is running standalone, then pop up an error dialog and call the \"Exit\" message."
                n170 = call <vilib>:"Simple Error Handler.vi"("error in (no error)"=w391) -> ()  [unwired: 4 in, 5 out]
                n171 = call-poly <vilib>:"Delacor_lib_QMH_Enqueue Message (poly).vi"("Priority Message? (F)"=TRUE, "Message"="Exit", "Message Queue in"=w390) -> ("error out"=w392:errorcluster)  [unwired: 7 in, 1 out]
              }
              frame True {
                # "If the module was launched externally, calling the Error Reported broadcast VI is the only action performed by the \"Error\" message. The module's caller can then process the error appropriately."
              }
            }
            n172 = Merge Errors(w384, w383) -> (w382:errorcluster)
            n173 = local write "error out"(w382) -> ()
          }
          frame "Exit" {
            w401 = 91  # 91: not all Exit messages will have an argument
            w403 = TRUE  # Stop the VI
            # "Release the message queue reference"
            # "Exit - Exit the application."
            n174 = Variant To Data(error in=w409, type=T4 {"Origin"="", "Exit via Stop Module Req?"=FALSE, "Wait for Module to stop?"=FALSE} ("Stop Argument"), Variant=w402) -> (data=w399:T4, error out=w405:errorcluster)
            n175 = call <vilib>:"Clear Errors.vi"("error in (no error)"=w405, "specific error code to clear (0: all)"=w401) -> ("error out"=w408:errorcluster)  [unwired: 4 in, 1 out]
            n176 = control-ref of="This VI"() -> (w398:refnum<vi>)
            n177 = Unbundle By Name(w395) -> ("DB.lvclass"=w394:refnum<class "DB.lvclass">)
            n178 = call "Handle Exit.vi"("Stop Argument"=w399, "Admin in"=w397, "VI reference"=w398) -> ("error out"=w396:errorcluster)  [unwired: 7 in, 1 out]
            n179 = call-dynamic "Delacor_lib_QMH_Release Message Queue.vi"("error in"=w408, "Message Queue"=w404) -> ("error out"=w407:errorcluster)  [unwired: 9 in]
            n180 = call-dynamic "Close DB Reference.vi"("error in (no error)"=w396, "DB in"=w394) -> ("error out"=w393:errorcluster)  [unwired: 8 in, 1 out]
            n181 = Merge Errors(w407, w393) -> (w406:errorcluster)
          }
          frame Default {
            # "'Default' case only runs if there is a message that isn't defined in any of the other cases.  Output a programming error."
            n182 = call "Module Name--constant.vi"() -> ("Module Name"=w410:string)  [unwired: 11 in]
            n183 = xnode "Error Ring"("parameter 0"=w411, "parameter 1"=w410) -> ("error out"=w415:errorcluster)
            n184 = Merge Errors(w413, w415) -> (w414:errorcluster)
          }
        }
        n185 = call-dynamic "Delacor_lib_QMH_Error Handler - Message Handling Loop.vi"("error in"=w171, "Message Queue in"=w161) -> ("dup error in"=w168:errorcluster)  [unwired: 8 in, 1 out]
      }
    }
    frame Error {
      # "Synchronize Caller Events.vi will inform Start Module.vi that the module has launched and will let the code calling Start Module.vi register for broadcasts and would permit the caller receive the broadcast that an error occurred at launch time."
      n186 = call-dynamic "Delacor_lib_QMH_Release Message Queue.vi"("error in"=w426, "Message Queue"=w424) -> ("error out"=w425:errorcluster)  [unwired: 9 in]
      n187 = call "Synchronize Caller Events.vi"("Singleton Module Admin in"=w427) -> ("error out"=w432:errorcluster)  [unwired: 9 in, 1 out]
      n188 = call "Module Name--constant.vi"() -> ("Module Name"=w430:string)  [unwired: 11 in]
      n189 = Format Into String(format string="An error occurred during initialization. %s is no longer running.", w430) -> (resulting string=w428:string)  [unwired: 2 in, 1 out]
      n190 = Merge Errors(w425, w432) -> (w433:errorcluster)
      n191 = call "Error Reported.vi"("Additional Information"=w428, "Error"=w433) -> ()  [unwired: 9 in, 1 out]
    }
  }
  n192 = Merge Errors(w15, w18) -> (w14:errorcluster)
  n193 = call "Close Module.vi"("error in (no error)"=w14, "Module Admin in"=w9) -> ("error out"=w16:errorcluster, "External Launch"=w2:bool, "Module Admin out"=w3:refnum<class "Delacor_lib_QMH_Module Admin.lvclass">)  [unwired: 7 in]
  n194 = Unregister For Events(event registration refnum=w8, error in=w16) -> (error out=w13:errorcluster)
  "error out" <- w13
  n195 = case "External Launch?" shown="True" w2 {
    tunnel: w13 -> [_ w434]
    frame False {
    }
    frame True {
      n196 = case shown="No Error" w434 {
        frame No Error {
          n197 = invoke class="VI" method="FP.Close"() -> ()  [unwired: 3 in, 3 out]
        }
        frame Error {
          n198 = invoke class="VI" method="FP.Open"("Activate"=TRUE ("Activate?")) -> ()  [unwired: 4 in, 5 out]
        }
      }
    }
  }
  n199 = local write "Module Admin"(w3) -> ()
